vi "Teardown.vi"(8 "error in":errorcluster, 11 "_Rename in":refnum<class "_Rename.lvclass">) -> (0 "error out":errorcluster)   [LabVIEW 2020, in "_Rename.lvlib" / "_Rename.lvclass"]
uses:
  _Rename.lvclass
  _Rename.lvclass/_Rename.ctl
  _Shared/Project Stuff/Project Stuff.lvclass
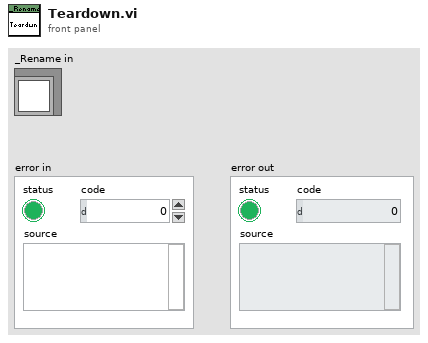
[diagram p1: front panel]
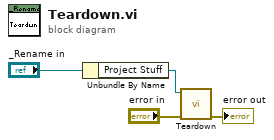
[diagram p0: block diagram]
diagram:
  n1 = Unbundle By Name("_Rename in") -> ("Project Stuff"=w1:refnum<class "Project Stuff.lvclass">)
  n2 = call "Teardown.vi"("Error in"="error in", "Project Stuff in"=w1) -> ("Error out"=→"error out":errorcluster)  [unwired: 9 in]
